vi "UMLEditor_TestFixXmlString.vi"() -> ()   [LabVIEW 2020]
panel:
  out "error out":errorcluster
  in  "Old":cluster{"Numeric":dbl, "Boolean":bool}
  in  "New":T1
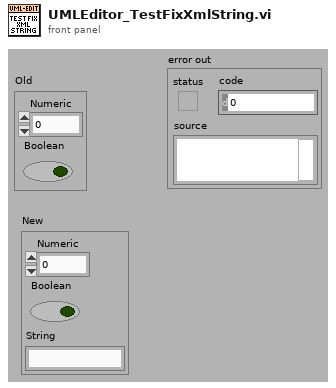
[diagram p1: front panel]
types:
  T1 = cluster{"Numeric":dbl, "Boolean":bool, "String":string}
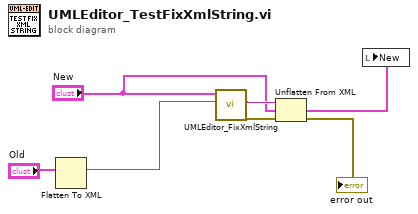
[diagram p0: block diagram]
diagram:
  n1 = Flatten To XML(6:"Old") -> (2:w6:string)
  n2 = call <resource>:"UMLEditor_FixXmlString.vi"("XML String"=w6, "CurrentCluster"="New") -> ("error out"=w2:errorcluster, "XML String"=w5:string)  [unwired: 8 in]
  n3 = Unflatten From XML(xml string=w5, type="New", error in (no error)=w2) -> (value=w3:T1, error out=→"error out":errorcluster)
  n4 = local write "New"(w3) -> ()
